vi "StopAll.vi"   [LabVIEW 2018]
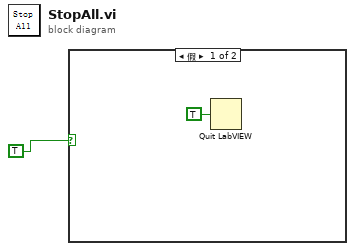
[diagram p0: block diagram]
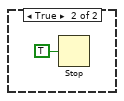
[diagram p2: hidden frame]
diagram:
  n1 = case shown="假" TRUE {
    frame False {
      n2 = Quit LabVIEW(quit? (T)=TRUE ("退出？(T)")) -> ()
    }
    frame True {
      n3 = Stop(stop? (T)=TRUE ("停止？(T)")) -> ()
    }
  }
